vi "Test Reset.vi"(8 "error in (no error)":errorcluster, 11 "Debug State Analyzer Test In":refnum<class "Debug State Analyzer Test.lvclass">) -> (0 "error out":errorcluster, 3 "Debug State Analyzer Test Out":refnum<class "Debug State Analyzer Test.lvclass">)   [LabVIEW 2020, in "Debug State Analyzer Test.lvclass"]
uses:
  Debug State Analyzer Test.lvclass
  Debug State Analyzer Test.lvclass/Debug State Analyzer Test.ctl
  01074fa8-ee8a-411d-bc8b-fc92c4f90959.vi
  source/State Analyzer/Debug State Analyzer.lvclass
  source/Debug Data/Raw Debug Data.ctl
  source/Debug Data/Debug Data.lvclass
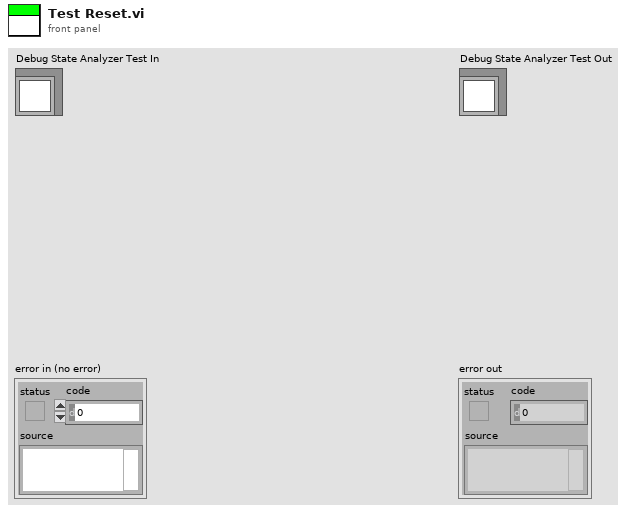
[diagram p1: front panel]
types:
  T1 = typedef "Debug Data.lvclass/Raw Debug Data.ctl" = cluster{"Action":string, "Call Chain":string, "Process":string, "Message":string, "Message Data":variant, "Time":dbl}
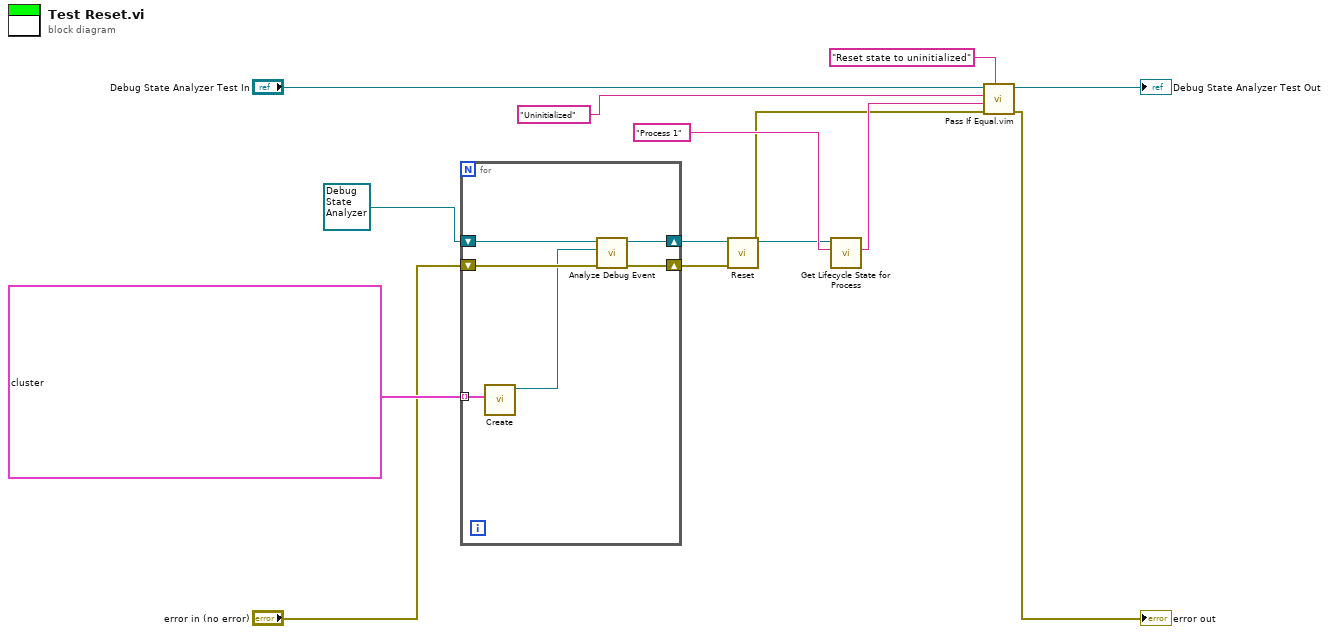
[diagram p0: block diagram]
diagram:
  n1 = for {
    tunnel: T1[] [{"Action"="Send", "Call Chain"="Test.vi:123456", "Process"="Process 1", "Message"="Init", "Message Data"=variant, "Time"=0.0}, {"Action"="Receive", "Call Chain"="TF.lvlib:Process.lvclass:Handle Messages.vi:1960001", "Process"="Process 1", "Message"="Init", "Message Data"=variant, "Time"=0.0}, {"Action"="Send", "Call Chain"="Test.vi", "Process"="Process 1", "Message"="Start", "Message Data"=variant, "Time"=0.0}, {"Action"="Receive", "Call Chain"="Test.vi", "Process"="Process 1", "Message"="Start", "Message Data"=variant, "Time"=0.0}, {"Action"="Send", "Call Chain"="Test.vi", "Process"="Process 1", "Message"="Stop", "Message Data"=variant, "Time"=0.0}, {"Action"="Receive", "Call Chain"="Test.vi", "Process"="Process 1", "Message"="Stop", "Message Data"=variant, "Time"=0.0}, {"Action"="Send", "Call Chain"="Test.vi", "Process"="Process 1", "Message"="Finish", "Message Data"=variant, "Time"=0.0}, {"Action"="Receive", "Call Chain"="Test.vi", "Process"="Process 1", "Message"="Finish", "Message Data"=variant, "Time"=0.0}] ("Debug Data Cluster") -> [w20] mode=indexing
    shift-right: [w18] -> w2
    shift-left: refnum<class "Debug State Analyzer.lvclass"> refnum ("Debug State Analyzer in") -> [w19]
    shift-right: [w16] -> w5
    shift-left: "error in (no error)" -> [w17]
    n2 = call "Create.vi"("Debug Data Cluster"=w20) -> ("Debug Data out"=w15:refnum<class "Debug Data.lvclass">)  [unwired: 9 in, 1 out]
    n3 = call "Analyze Debug Event.vi"("error in (no error)"=w17, "Debug Data.lvclass"=w15, "Debug State Analyzer In"=w19) -> ("error out"=w16:errorcluster, "Debug State Analyzer Out"=w18:refnum<class "Debug State Analyzer.lvclass">)  [unwired: 7 in]
  }
  n4 = call "Reset.vi"("error in (no error)"=w5, "Debug State Analyzer in"=w2) -> ("error out"=w3:errorcluster, "Debug State Analyzer out"=w1:refnum<class "Debug State Analyzer.lvclass">)  [unwired: 8 in]
  n5 = call "Get Lifecycle State for Process.vi"("Process"="Process 1", "Debug State Analyzer In"=w1) -> ("Lifecycle State"=w6:string)  [unwired: 8 in, 1 out]
  n6 = call "Pass If Equal.vim"("Description"="Reset state to uninitialized", "error in (no error)"=w3, "Actual"=w6, "Expected"="Uninitialized", "LUnit Test Case In"="Debug State Analyzer Test In") -> ("error out"=→"error out":errorcluster, "LUnit Test Case Out"=→"Debug State Analyzer Test Out":refnum<class "Debug State Analyzer Test.lvclass">)  [unwired: 5 in]
